vi "RPN.vi"(0 "Input stack\n(tokenized)":string[](array[string])) -> (1 "Output Queue":string[](array[string]), 2 "Errors?":string)   [LabVIEW 2012]
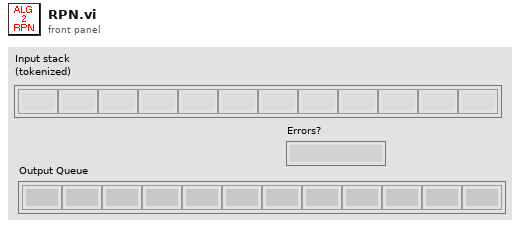
[diagram p1: front panel]
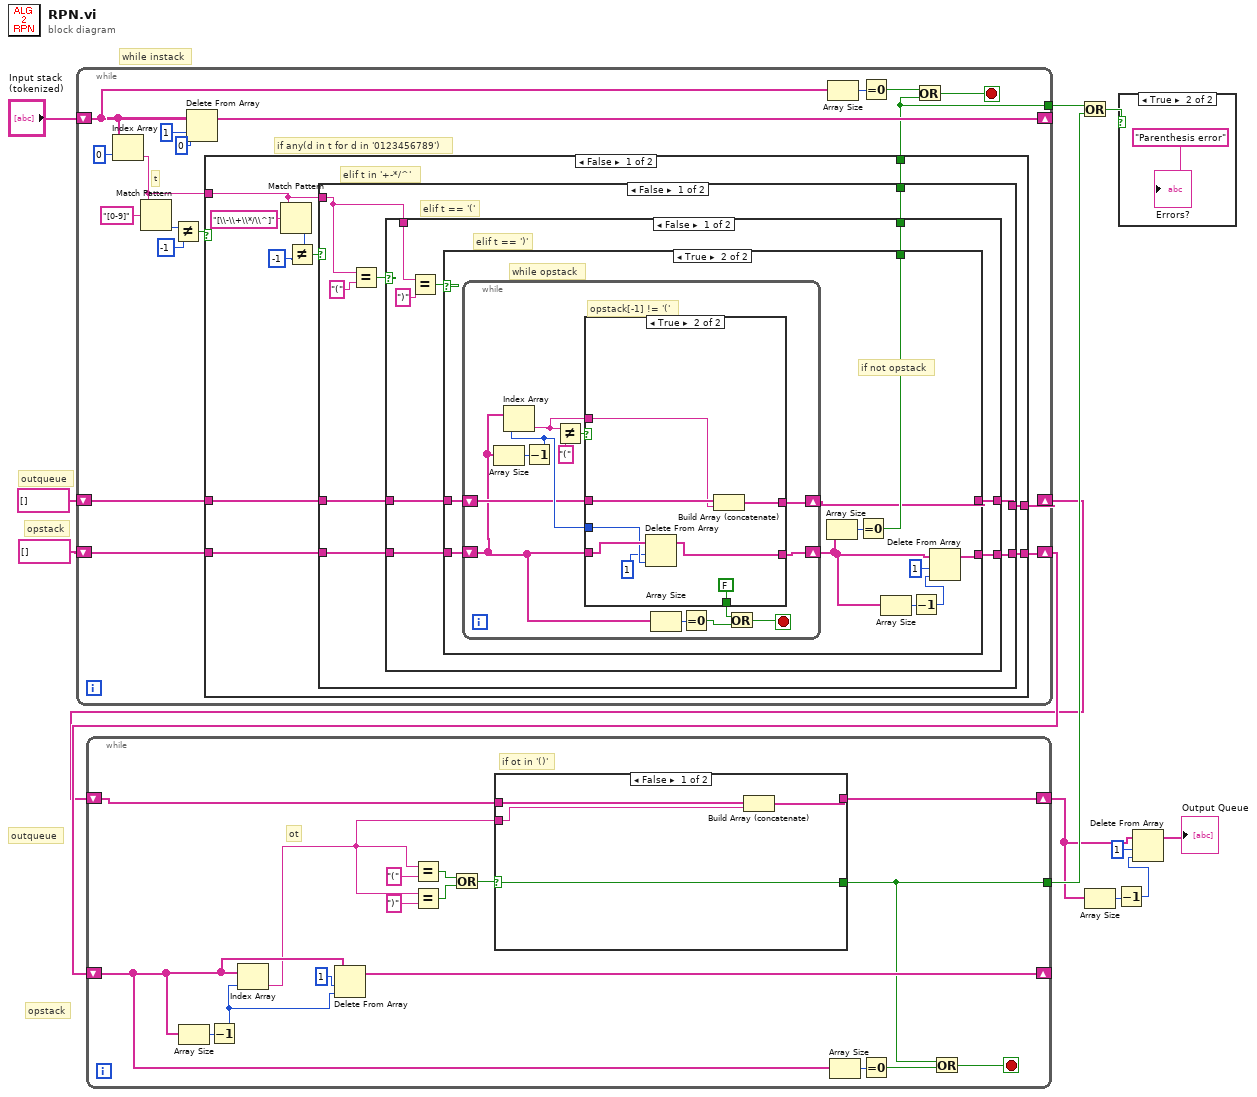
[diagram p0: block diagram]
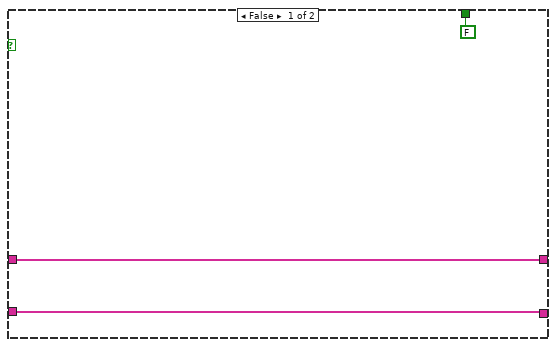
[diagram p4: hidden frame]
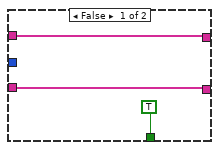
[diagram p5: hidden frame]
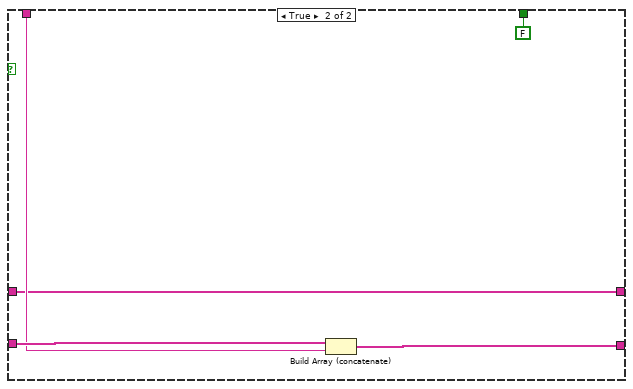
[diagram p6: hidden frame]
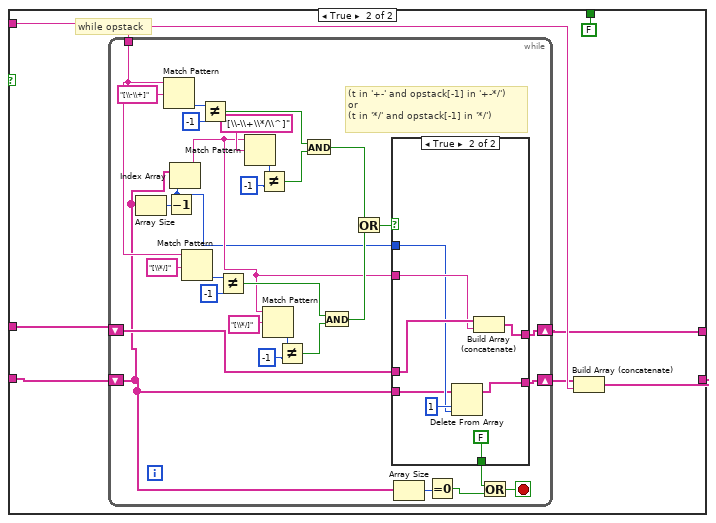
[diagram p7: hidden frame]
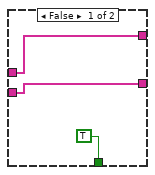
[diagram p8: hidden frame]
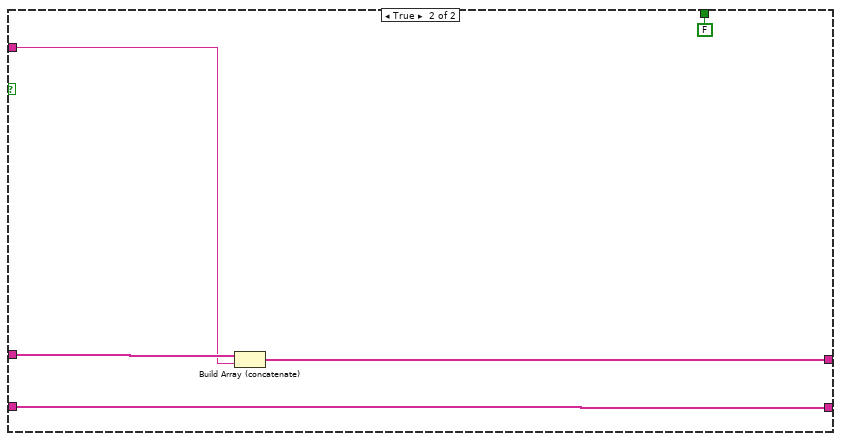
[diagram p9: hidden frame]
diagram:
  # "opstack"
  # "outqueue"
  # "while instack"
  # "opstack"
  # "outqueue"
  n1 = while {
    shift-right: [w24] -> w6
    shift-left: string[] [] -> [w25]
    shift-right: [w19] -> w10
    shift-left: string[] [] -> [w20]
    shift-right: [w28] -> _
    shift-left: "Input stack\n(tokenized)" -> [w16]
    tunnel: [w15] -> w8
    stop <- w18 stop-if-true
    # "t"
    # "if any(d in t for d in '0123456789')"
    n2 = Index Array(array=w16, index=0) -> (element=w14:string)
    n3 = Match Pattern(string=w14, regular expression="[0-9]") -> (offset past match=w23:i32)  [unwired: 1 in, 3 out]
    n4 = Not Equal?(x=w23, y=-1) -> (x != y?=w21:bool)
    n5 = Delete From Array(array=w16, length=1, index=0) -> (array with subset deleted=w28:string[])  [unwired: 1 out]
    n6 = case shown="False" w21 {
      tunnel: w25 -> [w35 w153]
      tunnel: [w34 w152] -> w24
      tunnel: w14 -> [w40 w151]
      tunnel: w20 -> [w36 w150]
      tunnel: [w33 w150] -> w19
      tunnel: [w32 FALSE] -> w15
      frame False {
        # "elif t in '+-*/^'"
        n7 = Match Pattern(string=w40, regular expression="[\\-\\+\\*/\\^]") -> (offset past match=w38:i32)  [unwired: 1 in, 3 out]
        n8 = Not Equal?(x=w38, y=-1) -> (x != y?=w39:bool)
        n9 = case shown="False" w39 {
          tunnel: w40 -> [w45 w105]
          tunnel: w36 -> [w47 w103]
          tunnel: w35 -> [w46 w102]
          tunnel: [w43 w101] -> w34
          tunnel: [w44 w106] -> w33
          tunnel: [w42 FALSE] -> w32
          frame False {
            # "elif t == '('"
            n10 = Equal?(x=w45, y="(") -> (x = y?=w48:bool)
            n11 = case shown="False" w48 {
              tunnel: w47 -> [w53 w99]
              tunnel: w46 -> [w54 w96]
              tunnel: w45 -> [w56 w98]
              tunnel: [w52 w97] -> w44
              tunnel: [w51 w96] -> w43
              tunnel: [w50 FALSE] -> w42
              frame False {
                # "elif t == ')'"
                n12 = Equal?(x=w56, y=")") -> (x = y?=w55:bool)
                n13 = case shown="True" w55 {
                  tunnel: w54 -> [w60 w63]
                  tunnel: w53 -> [w59 w64]
                  tunnel: [w59 w66] -> w52
                  tunnel: [w60 w62] -> w51
                  tunnel: [FALSE w65] -> w50
                  frame False {
                  }
                  frame True {
                    # "if not opstack"
                    # "while opstack"
                    n14 = while {
                      shift-right: [w71] -> w62
                      shift-left: w63 -> [w74]
                      shift-right: [w72] -> w61
                      shift-left: w64 -> [w73]
                      stop <- w78 stop-if-true
                      # "opstack[-1] != '('"
                      n15 = Array Size(array=w73) -> (size(s)=w82:i32)
                      n16 = Decrement(x=w82) -> (x-1=w79:i32)
                      n17 = Index Array(array=w73, index=w79) -> (element=w75:string)
                      n18 = Not Equal?(x=w75, y="(") -> (x != y?=w80:bool)
                      n19 = case shown="True" w80 {
                        tunnel: w74 -> [w84 w88]
                        tunnel: w73 -> [w85 w94]
                        tunnel: w79 -> [_ w93]
                        tunnel: [w85 w91] -> w72
                        tunnel: [w84 w90] -> w71
                        tunnel: [TRUE FALSE] -> w76
                        tunnel: w75 -> [_ w87]
                        frame False {
                        }
                        frame True {
                          n20 = Delete From Array(array=w94, length=1, index=w93) -> (array with subset deleted=w91:string[])  [unwired: 1 out]
                          n21 = Build Array (concatenate)(w88, w87) -> (w90:string[])
                        }
                      }
                      n22 = Array Size(array=w73) -> (size(s)=w83:i32)
                      n23 = Equal To 0?(x=w83) -> (x = 0?=w77:bool)
                      n24 = Or(x=w76, y=w77) -> (x .or. y?=w78:bool)
                    }
                    n25 = Array Size(array=w61) -> (size(s)=w70:i32)
                    n26 = Equal To 0?(x=w70) -> (x = 0?=w65:bool)
                    n27 = Array Size(array=w61) -> (size(s)=w69:i32)
                    n28 = Decrement(x=w69) -> (x-1=w67:i32)
                    n29 = Delete From Array(array=w61, length=1, index=w67) -> (array with subset deleted=w66:string[])  [unwired: 1 out]
                  }
                }
              }
              frame True {
                n30 = Build Array (concatenate)(w99, w98) -> (w97:string[])
              }
            }
          }
          frame True {
            # "while opstack"
            n31 = while {
              tunnel: w105 -> [w114]
              shift-right: [w108] -> w101
              shift-left: w102 -> [w110]
              shift-right: [w107] -> w100
              shift-left: w103 -> [w109]
              stop <- w113 stop-if-true
              # "(t in '+-' and opstack[-1] in '+-*/')\nor\n(t in '*/' and opstack[-1] in '*/')"
              n32 = Array Size(array=w109) -> (size(s)=w136:i32)
              n33 = Match Pattern(string=w114, regular expression="[\\-\\+]") -> (offset past match=w135:i32)  [unwired: 1 in, 3 out]
              n34 = Decrement(x=w136) -> (x-1=w117:i32)
              n35 = Index Array(array=w109, index=w117) -> (element=w118:string)
              n36 = Match Pattern(string=w114, regular expression="[\\*/]") -> (offset past match=w128:i32)  [unwired: 1 in, 3 out]
              n37 = Not Equal?(x=w135, y=-1) -> (x != y?=w130:bool)
              n38 = Not Equal?(x=w128, y=-1) -> (x != y?=w123:bool)
              n39 = Match Pattern(string=w118, regular expression="[\\-\\+\\*/\\^]") -> (offset past match=w133:i32)  [unwired: 1 in, 3 out]
              n40 = Not Equal?(x=w133, y=-1) -> (x != y?=w129:bool)
              n41 = Match Pattern(string=w118, regular expression="[\\*/]") -> (offset past match=w126:i32)  [unwired: 1 in, 3 out]
              n42 = Not Equal?(x=w126, y=-1) -> (x != y?=w122:bool)
              n43 = And(x=w130, y=w129) -> (x .and. y?=w121:bool)
              n44 = And(x=w123, y=w122) -> (x .and. y?=w120:bool)
              n45 = Or(x=w121, y=w120) -> (x .or. y?=w119:bool)
              n46 = case shown="True" w119 {
                tunnel: w110 -> [w139 w148]
                tunnel: [w139 w147] -> w108
                tunnel: w118 -> [_ w146]
                tunnel: w117 -> [_ w144]
                tunnel: w109 -> [w140 w143]
                tunnel: [w140 w142] -> w107
                tunnel: [TRUE FALSE] -> w111
                frame False {
                }
                frame True {
                  n47 = Delete From Array(array=w143, length=1, index=w144) -> (array with subset deleted=w142:string[])  [unwired: 1 out]
                  n48 = Build Array (concatenate)(w148, w146) -> (w147:string[])
                }
              }
              n49 = Array Size(array=w109) -> (size(s)=w137:i32)
              n50 = Equal To 0?(x=w137) -> (x = 0?=w112:bool)
              n51 = Or(x=w111, y=w112) -> (x .or. y?=w113:bool)
            }
            n52 = Build Array (concatenate)(w100, w105) -> (w106:string[])
          }
        }
      }
      frame True {
        n53 = Build Array (concatenate)(w153, w151) -> (w152:string[])
      }
    }
    n54 = Array Size(array=w16) -> (size(s)=w31:i32)
    n55 = Equal To 0?(x=w31) -> (x = 0?=w17:bool)
    n56 = Or(x=w17, y=w15) -> (x .or. y?=w18:bool)
  }
  n57 = while {
    shift-right: [w161] -> w5
    shift-left: w6 -> [w162]
    shift-right: [w163] -> _
    shift-left: w10 -> [w166]
    tunnel: [w160] -> w7
    stop <- w168 stop-if-true
    # "if ot in '()'"
    # "ot"
    n58 = Array Size(array=w166) -> (size(s)=w167:i32)
    n59 = Decrement(x=w167) -> (x-1=w165:i32)
    n60 = Index Array(array=w166, index=w165) -> (element=w155:string)
    n61 = Delete From Array(array=w166, length=1, index=w165) -> (array with subset deleted=w163:string[])  [unwired: 1 out]
    n62 = Equal?(x=w155, y="(") -> (x = y?=w158:bool)
    n63 = Equal?(x=w155, y=")") -> (x = y?=w157:bool)
    n64 = Or(x=w158, y=w157) -> (x .or. y?=w159:bool)
    n65 = case shown="False" w159 {
      selector: w159 -> [w174 w176]
      tunnel: w162 -> [w173 w175]
      tunnel: [w172 w175] -> w161
      tunnel: w155 -> [w171 _]
      tunnel: [w174 w176] -> w160
      frame False {
        n66 = Build Array (concatenate)(w173, w171) -> (w172:string[])
      }
      frame True {
      }
    }
    n67 = Array Size(array=w166) -> (size(s)=w170:i32)
    n68 = Equal To 0?(x=w170) -> (x = 0?=w169:bool)
    n69 = Or(x=w160, y=w169) -> (x .or. y?=w168:bool)
  }
  n70 = Or(x=w8, y=w7) -> (x .or. y?=w9:bool)
  n71 = Array Size(array=w5) -> (size(s)=w1:i32)
  n72 = Decrement(x=w1) -> (x-1=w4:i32)
  n73 = case shown="True" w9 {
    frame False {
    }
    frame True {
      "Errors?" <- "Parenthesis error" ("String")
    }
  }
  n74 = Delete From Array(array=w5, length=1, index=w4) -> (array with subset deleted=→"Output Queue":string[])  [unwired: 1 out]
